vi "Create_Object.vi"(8 "error in (no error)":errorcluster, 9 "Block Diagram in":T1, 10 "owner refnum":variant, 11 "Constant in":refnum<class "Constant.lvclass">) -> (0 "error out":errorcluster, 1 "Block Diagram Out":T1, 3 "Constant out":refnum<class "Constant.lvclass">)   [LabVIEW 2025, in "Constant.lvclass"]
uses:
  Constant.lvclass
  C:/Users/mrjak/Documents/GitHub/LVGPT/LabVIEW/VIs/Classes/Node/Node.lvclass
  Controls/bd.ctl
  Node.lvclass
  Controls/wire.ctl
  Controls/Terminal.ctl
  Node.lvclass/Node.ctl
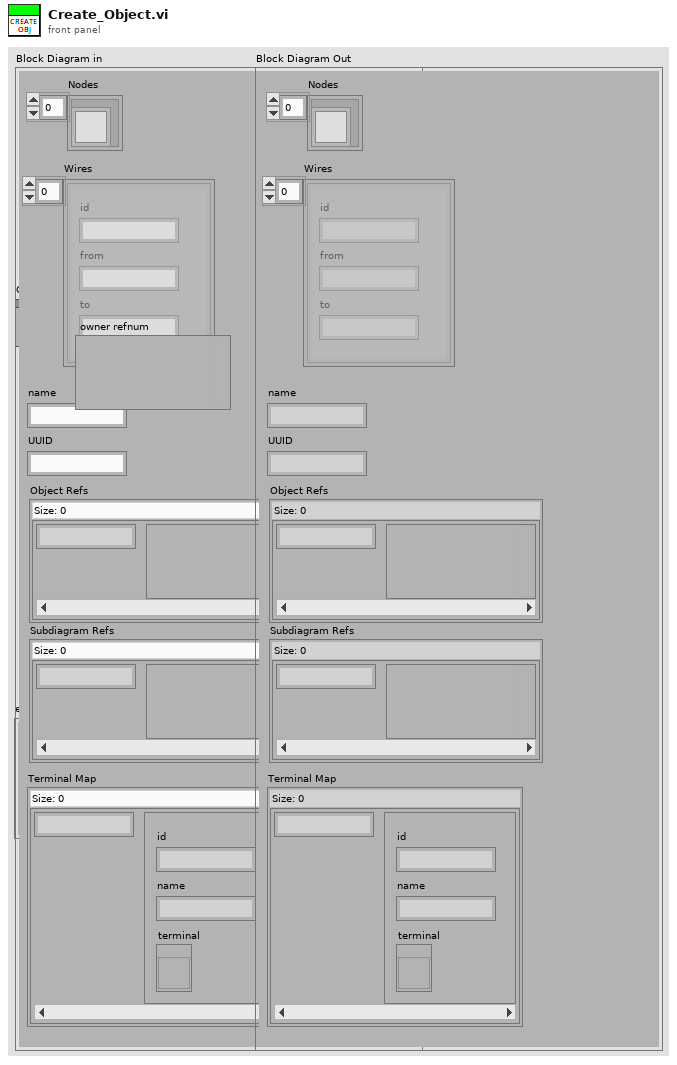
[diagram p1: front panel]
types:
  T1 = typedef "bd.ctl" = cluster{"Nodes":refnum<class "Node.lvclass">[], "Wires":T2[], "name":string, "UUID":string, "Object Refs":map{string, variant}, "Subdiagram Refs":map{string, variant}, "Terminal Map":map{string, T3}}
  T2 = typedef "wire.ctl" = cluster{"id":string, "from":string, "to":string}
  T3 = typedef "Terminal.ctl" = cluster{"id":string, "name":string, "terminal":refnum<vi>}
  T4 = typedef "LVPointTypeDef.ctl" = cluster{"Horizontal":i16, "Vertical":i16}
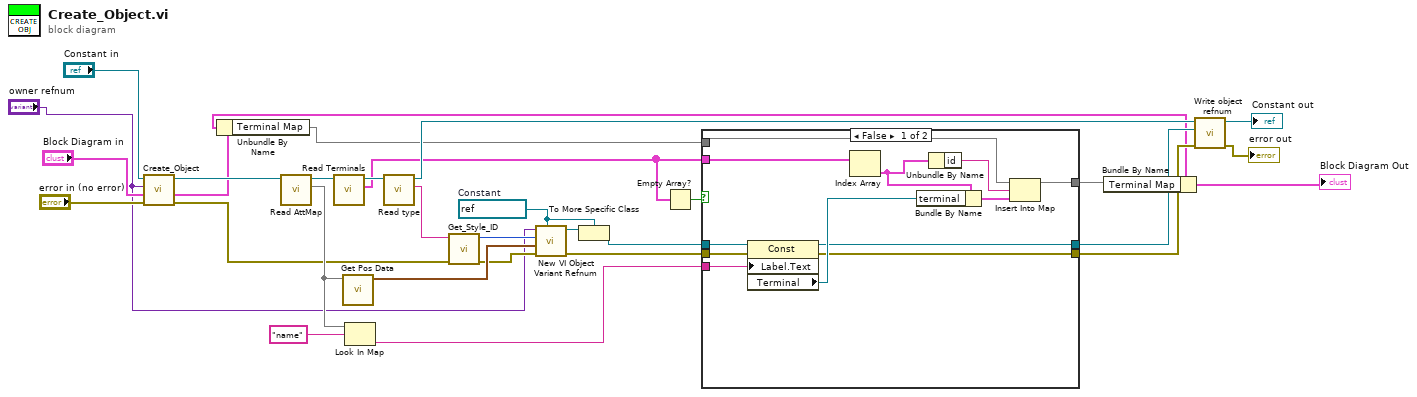
[diagram p0: block diagram]
diagram:
  w7 = refnum<vi> refnum  # Constant
  n1 = call-parent "Create_Object.vi"("error in (no error)"="error in (no error)", "Block Diagram in"="Block Diagram in", "owner refnum"="owner refnum", "Node in"="Constant in") -> ("error out"=w18:errorcluster, "Block Diagram Out"=w3:T1, "Node out"=w22:refnum<class "Constant.lvclass">)  [unwired: 5 in]
  n2 = Unbundle By Name(w3) -> ("Terminal Map"=w4:map{string, T3})
  n3 = call "Read AttMap.vi"("Node in"=w22) -> ("AttMap"=w23:map{string, string}, "Node out"=w27:refnum<class "Constant.lvclass">)  [unwired: 8 in, 1 out]
  n4 = call "Read Terminals.vi"("Node in"=w27) -> ("Terminals"=w5:T3[], "Node out"=w26:refnum<class "Constant.lvclass">)  [unwired: 8 in, 1 out]
  n5 = call "Get Pos Data.vi"("AttMap"=w23) -> ("Position"=w24:T4)  [unwired: 10 in]
  n6 = Look In Map(map=w23, key="name") -> (value=w10:string)  [unwired: 1 in, 1 out]
  n7 = call "Read type.vi"("Node in"=w26) -> ("type"=w20:string, "Node out"=w15:refnum<class "Constant.lvclass">)  [unwired: 8 in, 1 out]
  n8 = call "Get_Style_ID.vi"("error in (no error)"=w18, "Style"=w20) -> ("error out"=w19:errorcluster, "style"=w21:i32)  [unwired: 7 in, 1 out]
  n9 = call "New VI Object Variant Refnum.vi"("vi object class"=w7, "error in (no error)"=w19, "location"=w24, "style"=w21, "owner refnum"="owner refnum") -> ("error out"=w16:errorcluster, "object refnum"=w17:refnum<vi>)  [unwired: 5 in]
  n10 = To More Specific Class(target class=w7, reference=w17) -> (specific class reference=w8:refnum<vi>)  [unwired: 1 in, 1 out]
  n11 = Empty Array?(array=w5) -> (empty?=w6:bool)
  n12 = case shown="False" w6 {
    tunnel: w5 -> [w39 _]
    tunnel: w4 -> [w38 w43]
    tunnel: w16 -> [w37 w44]
    tunnel: [w35 w43] -> w2
    tunnel: [w34 w45] -> w14
    tunnel: [w33 w44] -> w13
    tunnel: w10 -> [w32 _]
    tunnel: w8 -> [w31 w45]
    frame False {
      n13 = property class="Const"(reference=w31, error in=w37, "Label.Text"=w32) -> (reference out=w34:refnum<vi>, error out=w33:errorcluster, "Terminal"=w36:refnum<vi>)
      n14 = Index Array(array=w39) -> (element=w41:T3)  [unwired: 1 in]
      n15 = Bundle By Name(cluster=w41, "terminal"=w36) -> (w40:T3)
      n16 = Unbundle By Name(w41) -> ("id"=w42:string)
      n17 = Insert Into Map(map in=w38, key=w42, value=w40) -> (map out=w35:map{string, T3})  [unwired: 2 out]
    }
    frame True {
    }
  }
  n18 = Bundle By Name(cluster=w3, "Terminal Map"=w2) -> (→"Block Diagram Out":T1)
  n19 = call-dynamic "Write object refnum.vi"("error in (no error)"=w13, "object refnum"=w14, "Node in"=w15) -> ("error out"=→"error out":errorcluster, "Node out"=→"Constant out":refnum<class "Constant.lvclass">)  [unwired: 7 in]
